vi "Autonomous Independent.vi"   [LabVIEW 2016]
doc: "This VI is called when autonomous begins, and will automatically be terminated when autonomous ends. You can carry out timed or sensor driven robot movement independently without needing to return to the caller."
uses:
  <vilib>/Rock Robotics/WPI/SafetyOutput/WPI_SafetyOutputConfigMenu.ctl
  <vilib>/Rock Robotics/WPI/Utilities/WPI_GetSetVariantRefNum.vi
  <vilib>/Rock Robotics/Network Tables/NT Read String.vi
  <vilib>/Rock Robotics/WPI/Ultrasonic/WPI_SonarMB1010AnalogRefNum Registry Get.vi
  <vilib>/Rock Robotics/Network Tables/NT Read Number.vi
  <vilib>/Rock Robotics/WPI/Ultrasonic/WPI_SonarMB1010AnalogGetRange.vi
  <vilib>/Rock Robotics/WPI/RobotDrive/WPI_RobotDriveArcadeDrive_Standard(NoSaturation).vi
  <vilib>/Rock Robotics/Network Tables/NT Write Numeric Array.vi
types:
  T1 = typedef "WPI_JoystickDevRef.ctl" = cluster{"Device":T2}
  T2 = typedef "WPI_JoystickDeviceEnum.ctl" = enum16{"USB 0", "USB 1", "USB 2", "USB 3", "USB 4", "USB 5"}
  T3 = typedef "WPI_SafetyOutputConfigMenu.ctl" = enum16{"Enable", "Disable"}
  T4 = typedef "WPI_SonarMB1010AnalogDeviceRef.ctl" = cluster{"AIDeviceRef":T5, "Scaling factor (V/in)":dbl, "Average Bits":u8}
  T5 = typedef "WPI_AnalogChannelDevRef.ctl" = cluster{"DevStatus":errorcluster, "Analog Channel":T6}
  T6 = typedef "FPGA_AIChannel.ctl" = enum8{"AI 0", "AI 1", "AI 2", "AI 3", "AI MXP 0", "AI MXP 1", "AI MXP 2", "AI MXP 3", "Invalid"}
  T7 = typedef "WPI_RobotDriveDevRef.ctl" = cluster{"DevStatus":errorcluster, "Motors[]":T8[], "Square Inputs":bool, "Max Output":dbl}
  T8 = typedef "WPI_MotorControlDeviceRef.ctl" = cluster{"DeviceStatus":errorcluster, "Type":T9, "PWM":cluster{"PWM Channel":T10, "DeadBand":T11}, "CAN":cluster{"Device Number":u8, "SetOutput VI Ref":variant, "GetOutput VI Ref":variant, "Enable VI Ref":variant, "Disable VI Ref":variant, "Data":variant}, "Invert":bool}
  T9 = typedef "WPI_MotorControlType.ctl" = enum16{"PWM", "CAN"}
  T10 = typedef "FPGA_DIOPWMChannel.ctl" = enum8{"PWM 0", "PWM 1", "PWM 2", "PWM 3", "PWM 4", "PWM 5", "PWM 6", "PWM 7", "PWM 8", "PWM 9", "PWM MXP 0", "PWM MXP 1", "PWM MXP 2", "PWM MXP 3", "PWM MXP 4", "PWM MXP 5", "PWM MXP 6", "PWM MXP 7", "PWM MXP 8", "PWM MXP 9", "Invalid"}
  T11 = typedef "WPI_PWMDeadband.ctl" = cluster{"Name":string, "maxPositivePwm":i32, "minPositivePwm":i32, "centerPwm":i32, "maxNegativePwm":i32, "minNegativePwm":i32, "angularRange":u16}
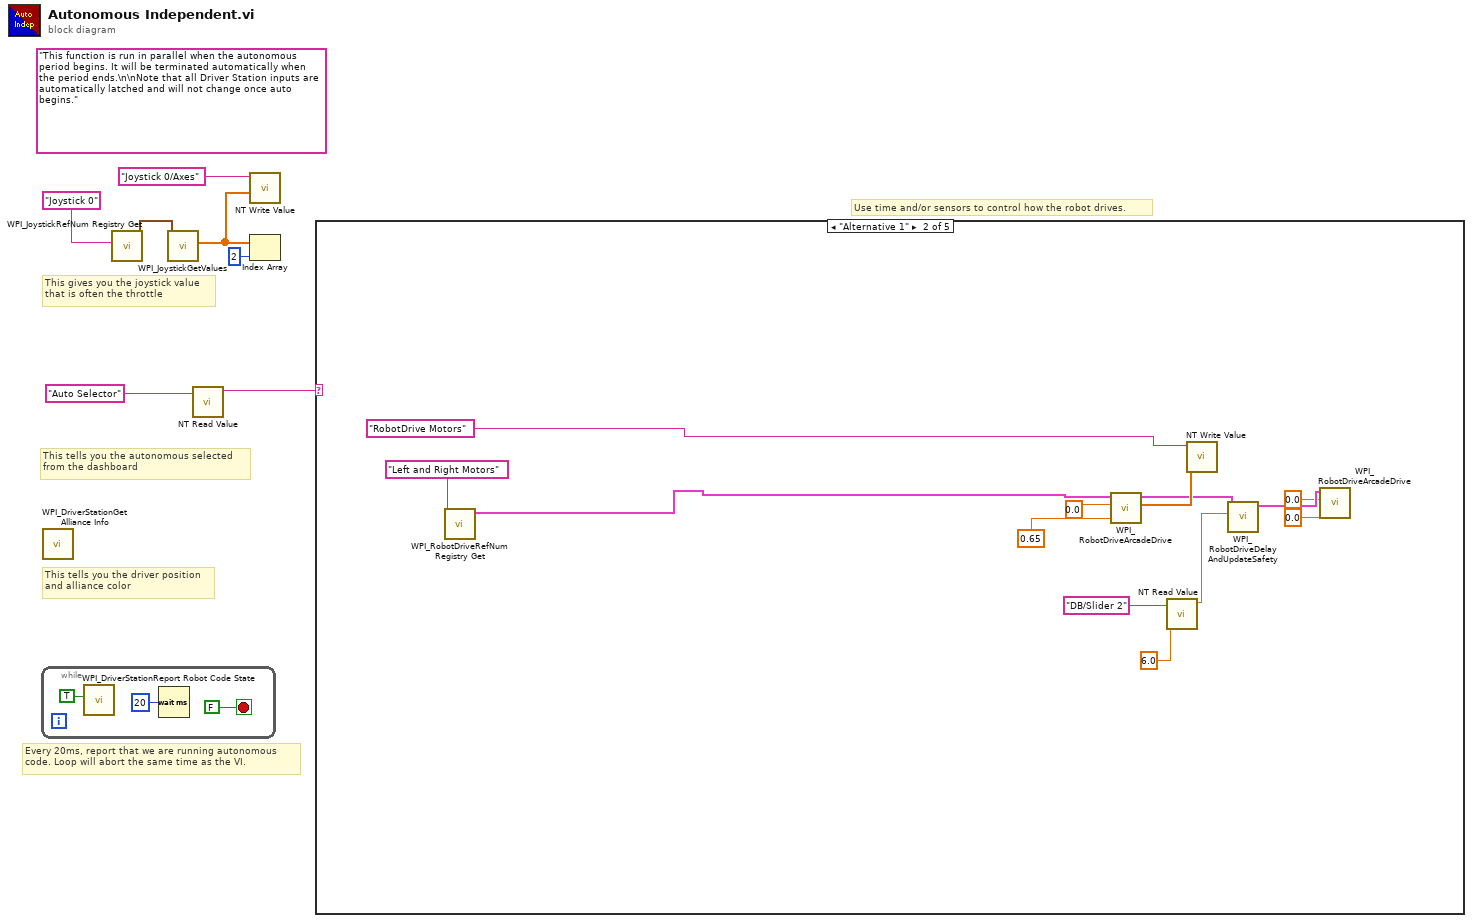
[diagram p0: block diagram]
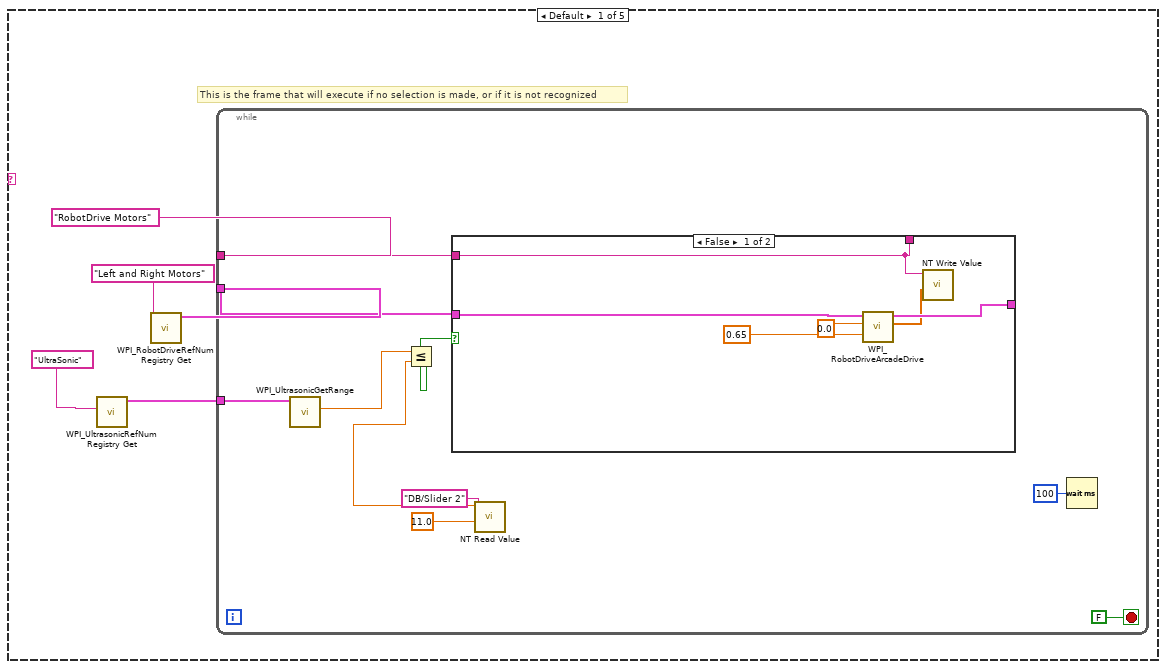
[diagram p2: hidden frame]
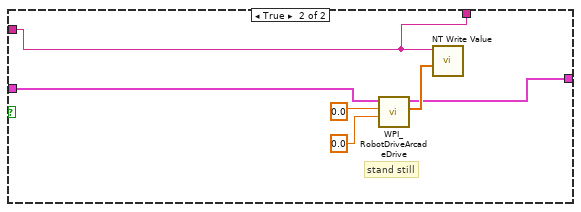
[diagram p3: hidden frame]
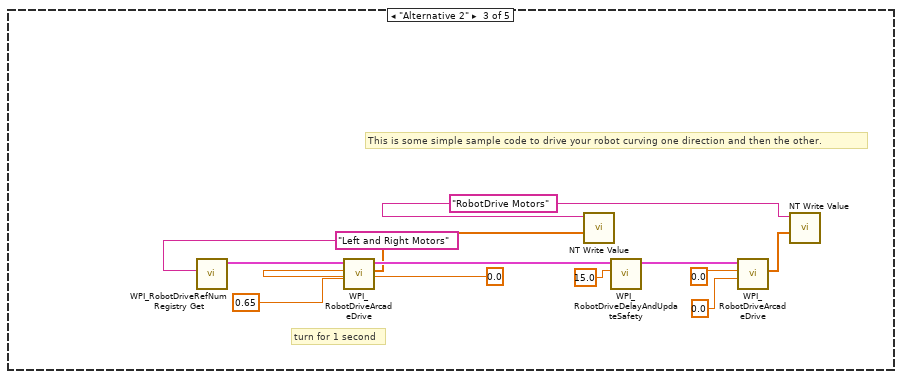
[diagram p4: hidden frame]
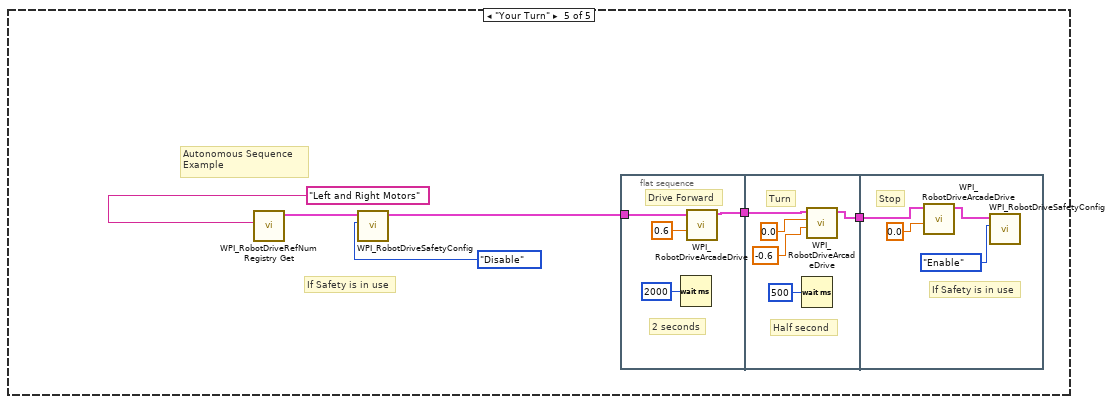
[diagram p6: hidden frame]
diagram:
  (unwired) "This function is run in parallel when the autonomous period begins. It will be terminated automatically when the period ends.\n\nNote that all Driver Station inputs are automatically latched and will not change once auto begins."
  # "This tells you the autonomous selected\nfrom the dashboard"
  # "Every 20ms, report that we are running autonomous\ncode. Loop will abort the same time as the VI."
  # "This gives you the joystick value\nthat is often the throttle"
  # "Use time and/or sensors to control how the robot drives."
  # "This tells you the driver position\nand alliance color"
  n1 = while {
    stop <- FALSE stop-if-true
    n2 = call <vilib>:"WPI_DriverStationReport Robot Code State.vi"("Autonomous"=TRUE) -> ()  [unwired: 10 in, 1 out]
    n3 = Wait (ms)(milliseconds to wait=u32 20) -> ()  [unwired: 1 out]
  }
  n4 = call <vilib>:"WPI_DriverStationGet Alliance Info.vi"() -> ()  [unwired: 12 out]
  n5 = call <vilib>:"WPI_JoystickRefNum Registry Get.vi"("refnum name"="Joystick 0") -> ("JoystickDevRef"=w6:T1)  [unwired: 1 in, 9 out]
  n6 = call <vilib>:"WPI_JoystickGetValues.vi"("JoystickDevRef"=w6) -> ("Axes"=w2:dbl[])  [unwired: 6 in, 4 out]
  n7 = call-poly <vilib>:"NT Read Value.vi"("Name"="Auto Selector") -> ("String"=w3:string)  [unwired: 9 in, 1 out]
  n8 = call-poly <vilib>:"NT Write Value.vi"("Numeric Array"=w2, "Name"="Joystick 0/Axes") -> ()  [unwired: 9 in, 1 out]
  n9 = Index Array(array=w2, index=2) -> ()  [unwired: 1 out]
  n10 = case shown="\"Alternative 1\"" w3 {
    frame Default {
      # "This is the frame that will execute if no selection is made, or if it is not recognized"
      n11 = call-poly <vilib>:"WPI_UltrasonicRefNum Registry Get.vi"("refnum name"="UltraSonic") -> ("SonarMB1010AnalogDevRef"=w11:T4)  [unwired: 9 in, 1 out]
      n12 = call <vilib>:"WPI_RobotDriveRefNum Registry Get.vi"("refnum name"="Left and Right Motors") -> ("RobotDriveDevRef"=w12:T7)  [unwired: 1 in, 9 out]
      n13 = while {
        tunnel: "RobotDrive Motors" ("Name") -> [w24]
        tunnel: w12 -> [w23]
        tunnel: w11 -> [w21]
        stop <- FALSE stop-if-true
        n14 = call-poly <vilib>:"WPI_UltrasonicGetRange.vi"("SonarMB1010AnalogDevRef"=w21) -> ("Distance"=w22:dbl)  [unwired: 8 in, 2 out]
        n15 = call-poly <vilib>:"NT Read Value.vi"("Default Value"=11.0, "Name"="DB/Slider 2") -> ("Numeric"=w16:dbl)  [unwired: 8 in, 1 out]
        n16 = Less Or Equal?(x=w22, y=w16) -> (x <= y?=w25:bool)
        n17 = case shown="False" w25 {
          tunnel: w24 -> [w30 w32]
          tunnel: [w30 w32] -> _
          tunnel: w23 -> [w29 w34]
          tunnel: [w28 w33] -> _
          frame False {
            n18 = call-poly <vilib>:"WPI_RobotDriveArcadeDrive.vi"("Y axis value"=0.65, "X axis value"=0.0, "RobotDriveDevRef"=w29) -> ("Motor Values"=w26:dbl[], "RobotDriveDevRef"=w28:T7)  [unwired: 1 in, 6 out]
            n19 = call-poly <vilib>:"NT Write Value.vi"("Numeric Array"=w26, "Name"=w30) -> ()  [unwired: 9 in, 1 out]
          }
          frame True {
            # "stand still"
            n20 = call-poly <vilib>:"WPI_RobotDriveArcadeDrive.vi"("Y axis value"=0.0 ("X axis value"), "X axis value"=0.0, "RobotDriveDevRef"=w34) -> ("Motor Values"=w37:dbl[], "RobotDriveDevRef"=w33:T7)  [unwired: 1 in, 6 out]
            n21 = call-poly <vilib>:"NT Write Value.vi"("Numeric Array"=w37, "Name"=w32) -> ()  [unwired: 9 in, 1 out]
          }
        }
        n22 = Wait (ms)(milliseconds to wait=u32 100) -> ()  [unwired: 1 out]
      }
    }
    frame "Alternative 1" {
      n23 = call <vilib>:"WPI_RobotDriveRefNum Registry Get.vi"("refnum name"="Left and Right Motors") -> ("RobotDriveDevRef"=w46:T7)  [unwired: 1 in, 9 out]
      n24 = call-poly <vilib>:"WPI_RobotDriveArcadeDrive.vi"("Y axis value"=0.65, "X axis value"=0.0, "RobotDriveDevRef"=w46) -> ("Motor Values"=w47:dbl[], "RobotDriveDevRef"=w44:T7)  [unwired: 1 in, 6 out]
      n25 = call-poly <vilib>:"NT Read Value.vi"("Default Value"=6.0, "Name"="DB/Slider 2") -> ("Numeric"=w40:dbl)  [unwired: 8 in, 1 out]
      n26 = call-poly <vilib>:"NT Write Value.vi"("Numeric Array"=w47, "Name"="RobotDrive Motors") -> ()  [unwired: 9 in, 1 out]
      n27 = call <vilib>:"WPI_RobotDriveDelayAndUpdateSafety.vi"("Delay (s)"=w40, "RobotDriveDevRef"=w44) -> ("RobotDriveDevRef 2"=w43:T7)  [unwired: 8 in, 1 out]
      n28 = call-poly <vilib>:"WPI_RobotDriveArcadeDrive.vi"("Y axis value"=0.0, "X axis value"=0.0, "RobotDriveDevRef"=w43) -> ()  [unwired: 1 in, 8 out]
    }
    frame "Alternative 2" {
      w53 = "RobotDrive Motors" ("Name")
      # "This is some simple sample code to drive your robot curving one direction and then the other."
      # "turn for 1 second"
      n29 = call <vilib>:"WPI_RobotDriveRefNum Registry Get.vi"("refnum name"="Left and Right Motors") -> ("RobotDriveDevRef"=w62:T7)  [unwired: 1 in, 9 out]
      n30 = call-poly <vilib>:"WPI_RobotDriveArcadeDrive.vi"("Y axis value"=0.65 ("Default Value"), "X axis value"=0.0, "RobotDriveDevRef"=w62) -> ("Motor Values"=w52:dbl[], "RobotDriveDevRef"=w58:T7)  [unwired: 1 in, 6 out]
      n31 = call-poly <vilib>:"NT Write Value.vi"("Numeric Array"=w52, "Name"=w53) -> ()  [unwired: 9 in, 1 out]
      n32 = call <vilib>:"WPI_RobotDriveDelayAndUpdateSafety.vi"("Delay (s)"=15.0, "RobotDriveDevRef"=w58) -> ("RobotDriveDevRef 2"=w59:T7)  [unwired: 8 in, 1 out]
      n33 = call-poly <vilib>:"WPI_RobotDriveArcadeDrive.vi"("Y axis value"=0.0 ("X axis value"), "X axis value"=0.0, "RobotDriveDevRef"=w59) -> ("Motor Values"=w54:dbl[])  [unwired: 1 in, 7 out]
      n34 = call-poly <vilib>:"NT Write Value.vi"("Numeric Array"=w54, "Name"=w53) -> ()  [unwired: 9 in, 1 out]
    }
    frame "Sonar Infused" {
    }
    frame "Your Turn" {
      # "If Safety is in use"
      # "Autonomous Sequence\nExample"
      n35 = call <vilib>:"WPI_RobotDriveRefNum Registry Get.vi"("refnum name"="Left and Right Motors") -> ("RobotDriveDevRef"=w65:T7)  [unwired: 9 in, 1 out]
      n36 = call <vilib>:"WPI_RobotDriveSafetyConfig.vi"("mode"=WPI_SafetyOutputConfigMenu."Disable", "RobotDriveDevRef"=w65) -> ("RobotDriveDevRef"=w64:T7)  [unwired: 8 in, 1 out]
      n37 = flat-sequence {
        tunnel: w64 -> [w70]
        tunnel: [w69] -> w68
        tunnel: [w76] -> w67
        tunnel: w68 -> [w75]
        tunnel: w67 -> [w79]
        frame #0 {
          # "2 seconds"
          # "Drive Forward"
          n38 = Wait (ms)(milliseconds to wait=u32 2000) -> ()  [unwired: 1 out]
          n39 = call-poly <vilib>:"WPI_RobotDriveArcadeDrive.vi"("Y axis value"=0.6 ("Left axis value"), "RobotDriveDevRef"=w70) -> ("RobotDriveDevRef"=w69:T7)  [unwired: 7 in, 2 out]
        }
        frame #1 {
          # "Half second"
          # "Turn"
          n40 = Wait (ms)(milliseconds to wait=u32 500) -> ()  [unwired: 1 out]
          n41 = call-poly <vilib>:"WPI_RobotDriveArcadeDrive.vi"("Y axis value"=-0.6 ("Right axis value"), "X axis value"=0.0 ("Left axis value"), "RobotDriveDevRef"=w75) -> ("RobotDriveDevRef"=w76:T7)  [unwired: 6 in, 2 out]
        }
        frame #2 {
          # "If Safety is in use"
          # "Stop"
          n42 = call-poly <vilib>:"WPI_RobotDriveArcadeDrive.vi"("Y axis value"=0.0 ("Left axis value"), "RobotDriveDevRef"=w79) -> ("RobotDriveDevRef"=w78:T7)  [unwired: 7 in, 2 out]
          n43 = call <vilib>:"WPI_RobotDriveSafetyConfig.vi"("mode"=WPI_SafetyOutputConfigMenu."Enable", "RobotDriveDevRef"=w78) -> ()  [unwired: 8 in, 2 out]
        }
      }
    }
  }
